vi "Add Property (Array).vi"(7 "Required?":bool, 8 "error in (no error)":errorcluster, 9 "Array Ref in":refnum<vi>, 11 "JSON Schema in":string) -> (0 "error out":errorcluster, 3 "JSON SChema out":string)   [LabVIEW 2020, in "JSON Schema Generator.lvlib"]
uses:
  JSON Schema Generator.lvlib
  <vilib>/JDP Science/JSONtext/LVClass Serializer/JSONtext LVClass Serializer.lvclass
  <vilib>/JDP Science/JSONtext/JSONtext.lvlib
  3b38040d-3c80-4d5d-94cc-ad2b8314f827.vi
  <vilib>/Utility/Data Type/NI_Data Type.lvlib
  <userlib>/_OpenG.lib/error/error.llb/openg_error.lvlib
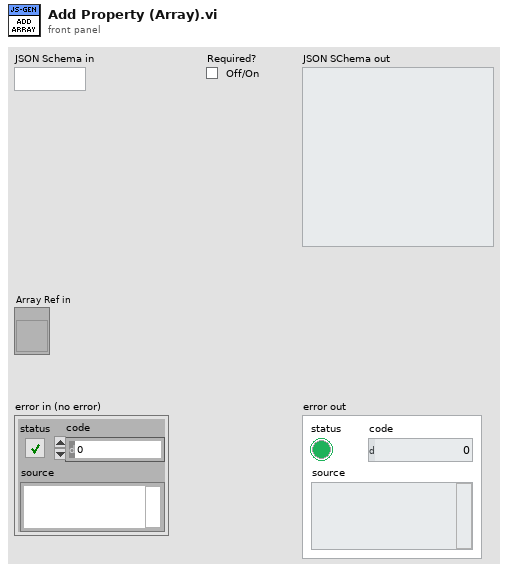
[diagram p1: front panel]
types:
  T1 = typedef "NI_Data Type.lvlib/Data Type.ctl" = enum8{"Invalid Type", "Void", "I8", "I16", "I32", "I64", "U8", "U16", "U32", "U64", "Single Float", "Double Float", "Extended Float", "Single Complex", "Double Complex", "Extended Complex", "Enum U8", "Enum U16", "Enum U32", "Enum U64", "Single Float With Unit", "Double Float With Unit", "Extended Float With Unit", "Single Complex with Unit", "Double Complex with Unit", "Extended Complex with Unit", "Boolean", "String", "Path", "Picture", "Tag", "Array", "Cluster", "Variant", "LV Variant", "Waveform", "Timestamp", "Digital Waveform", "Digital Data", "ExpressData", "Refnum", "External Data", "VI", "Poly VI", "LabVIEW Class Instance", "Fixed Point", "Set Collection", "Map Collection"}
  T2 = typedef "NI_Data Type.lvlib/Type Definition Info.ctl" = cluster{"Name":string, "Timestamp":u32}
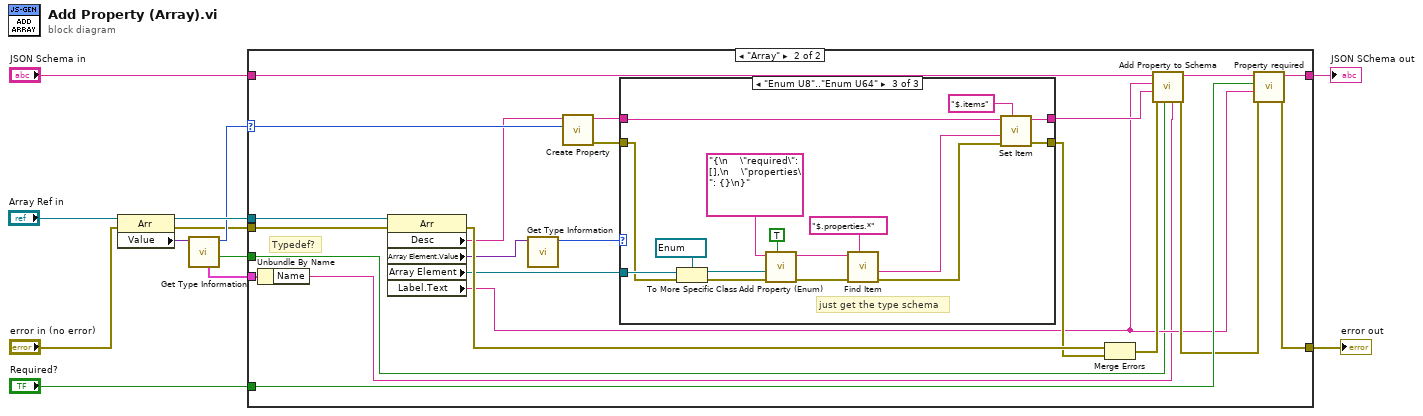
[diagram p0: block diagram]
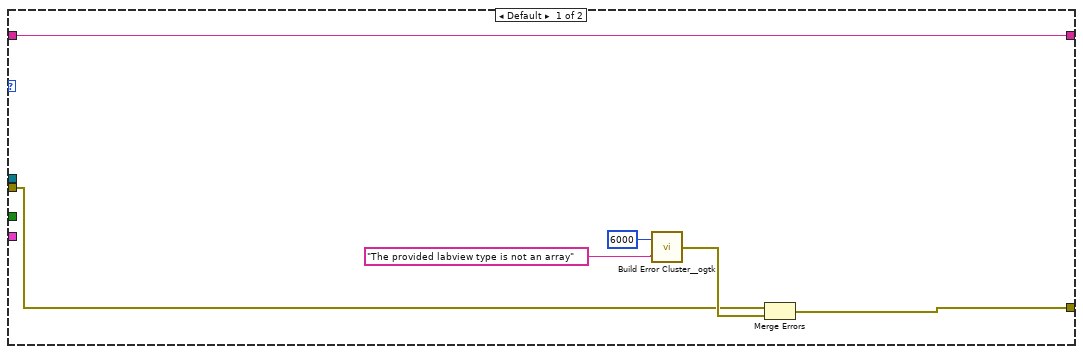
[diagram p2: hidden frame]
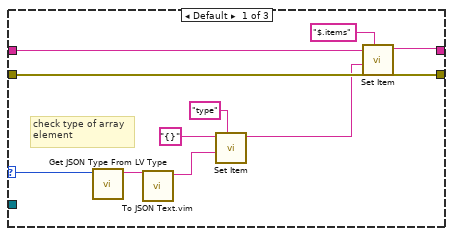
[diagram p3: hidden frame]
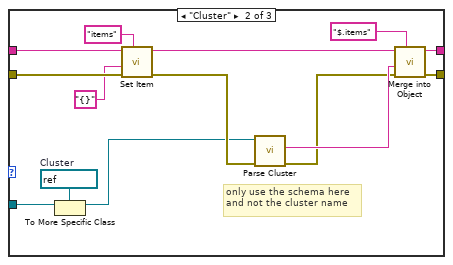
[diagram p4: hidden frame]
diagram:
  n1 = property class="Arr"(reference="Array Ref in", error in="error in (no error)") -> (reference out=w7:refnum<vi>, error out=w4:errorcluster, "Value"=w6:variant)
  n2 = call <vilib>:"Get Type Information.vi"("variant"=w6) -> ("type definition"=w2:bool, "type"=w5:T1, "type definition info"=w1:T2)  [unwired: 6 in, 2 out]
  n3 = case shown="\"Array\"" w5 {
    selector: w5 -> [_ w37]
    tunnel: [w18 w40] -> w12
    tunnel: "Required?" -> [_ w39]
    tunnel: [w16 w38] -> w10
    tunnel: "JSON Schema in" -> [w18 w35]
    tunnel: w7 -> [_ w31]
    tunnel: w4 -> [w13 w22]
    tunnel: w2 -> [_ w21]
    tunnel: w1 -> [_ w20]
    frame Default {
      n4 = call <userlib>:"Build Error Cluster__ogtk.vi"("String to Prepend to source (\"\")"="The provided labview type is not an array" ("String to Prepend to source (\"\")"), "code"=6000) -> ("error out"=w17:errorcluster)
      n5 = Merge Errors(w13, w17) -> (w16:errorcluster)
    }
    frame "Array" {
      # "Typedef?"
      n6 = Unbundle By Name(w20) -> ("Name"=w19:string)
      n7 = property class="Arr"(reference=w31, error in=w22) -> (error out=w41:errorcluster, "Desc"=w24:string, "Array Element.Value"=w32:variant, "Array Element"=w29:refnum<vi>, "Label.Text"=w23:string)  [unwired: 1 out]
      n8 = call <vilib>:"Get Type Information.vi"("variant"=w32) -> ("type"=w26:T1)  [unwired: 6 in, 4 out]
      n9 = call "Create Property.vi"("Labview Type"=w37, "Description"=w24) -> ("error out"=w28:errorcluster, "JSON Schema Property out"=w27:string)  [unwired: 8 in]
      n10 = case shown="\"Enum U8\"..\"Enum U64\"" w26 {
        selector: w26 -> [w47 _ _]
        tunnel: [w50 w66 w74] -> w30
        tunnel: w29 -> [_ w64 w69]
        tunnel: w28 -> [w52 w62 w67]
        tunnel: w27 -> [w51 w61 w72]
        tunnel: [w42 w58 w73] -> w25
        frame Default {
          # "check type of array\nelement"
          n11 = call "Get JSON Type From LV Type.vi"("Labview Datatype"=w47) -> ("JSON Schema Type"=w48:string)  [unwired: 9 in, 1 out]
          n12 = call "To JSON Text.vim"("Anything"=w48) -> ("<JSON>"=w49:string)  [unwired: 9 in, 1 out]
          n13 = call <vilib>:"Set Item.vi"("$Path or Item Name"="type", "JSON to Insert"=w49, "JSON"="{}") -> ("<JSON>"=w45:string)  [unwired: 5 in, 2 out]
          n14 = call <vilib>:"Set Item.vi"("$Path or Item Name"="$.items", "error in (no error)"=w52, "JSON to Insert"=w45, "JSON"=w51) -> ("error out"=w42:errorcluster, "<JSON>"=w50:string)  [unwired: 4 in, 1 out]
        }
        frame "Cluster" {
          w63 = refnum<vi> refnum  # Cluster
          # "only use the schema here\nand not the cluster name"
          n15 = To More Specific Class(target class=w63, reference=w64) -> (specific class reference=w53:refnum<vi>)  [unwired: 1 in, 1 out]
          n16 = call <vilib>:"Set Item.vi"("$Path or Item Name"="items", "error in (no error)"=w62, "JSON to Insert"="{}", "JSON"=w61) -> ("error out"=w55:errorcluster, "<JSON>"=w60:string)  [unwired: 4 in, 1 out]
          n17 = call "Parse Cluster.vi"("error in"=w55, "Cluster Refnum In"=w53) -> ("error out"=w54:errorcluster, "JSON ObjectSchema out"=w65:string)  [unwired: 5 in, 3 out]
          n18 = call <vilib>:"Merge into Object.vi"("$Path or Item Name"="$.items" ("string"), "error in (no error)"=w54, "JSON Object to Merge"=w65, "JSON"=w60) -> ("error out"=w58:errorcluster, "<JSON>"=w66:string)  [unwired: 5 in]
        }
        frame "Enum U8".."Enum U64" {
          # "just get the type schema"
          n19 = To More Specific Class(target class=refnum<vi> refnum ("Other Refnum"), reference=w69, error in=w67) -> (specific class reference=w80:refnum<vi>, error out=w68:errorcluster)
          n20 = call "Add Property (Enum).vi"("Required?"=TRUE, "error in (no error)"=w68, "Enum In"=w80, "JSON Schema in"="{\n    \"required\": [],\n    \"properties\": {}\n}" ("JSON")) -> ("error out"=w70:errorcluster, "JSON SChema out"=w71:string)  [unwired: 6 in]
          n21 = call <vilib>:"Find Item.vi"("$Path or Item Name"="$.properties.*", "error in (no error)"=w70, "JSON"=w71) -> ("error out"=w77:errorcluster, "<JSON>"=w76:string)  [unwired: 5 in, 2 out]
          n22 = call <vilib>:"Set Item.vi"("$Path or Item Name"="$.items", "error in (no error)"=w77, "JSON to Insert"=w76, "JSON"=w72) -> ("error out"=w73:errorcluster, "<JSON>"=w74:string)  [unwired: 4 in, 1 out]
        }
      }
      n23 = Merge Errors(w41, w25) -> (w33:errorcluster)
      n24 = call "Add Property to Schema.vi"("Typedef Name"=w19, "Typedef?"=w21, "error in"=w33, "JSON Schema Property in"=w30, "Property Name"=w23, "JSON Schema in"=w35) -> ("error out"=w34:errorcluster, "JSON Schema out"=w36:string)  [unwired: 4 in]
      n25 = call "Property required.vi"("error in (no error)"=w34, "Name"=w23, "Required?"=w39, "JSON Schema in"=w36) -> ("error out"=w38:errorcluster, "JSON Schema out"=w40:string)  [unwired: 6 in]
    }
  }
  "JSON SChema out" <- w12
  "error out" <- w10
